vi "Write Shared Approved File Path.vi"(8 "error in":errorcluster, 10 "Shared Approved File Path":path, 11 "Namer With Shared Approved File in":refnum<class "Namer With Shared Approved File.lvclass">) -> (0 "error out":errorcluster, 3 "Namer With Shared Approved File out":refnum<class "Namer With Shared Approved File.lvclass">)   [LabVIEW 2020, in "Approval Tests.lvlib" / "Namer With Shared Approved File.lvclass"]
uses:
  Namer With Shared Approved File.lvclass
  Namer With Shared Approved File.lvclass/Namer With Shared Approved File.ctl
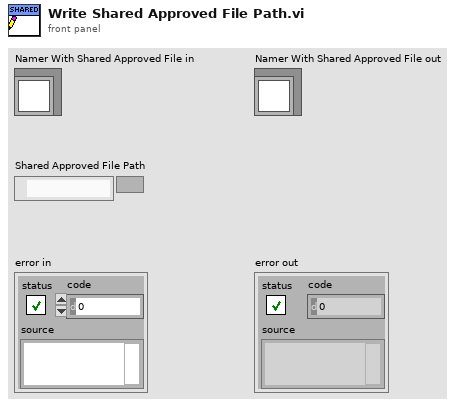
[diagram p1: front panel]
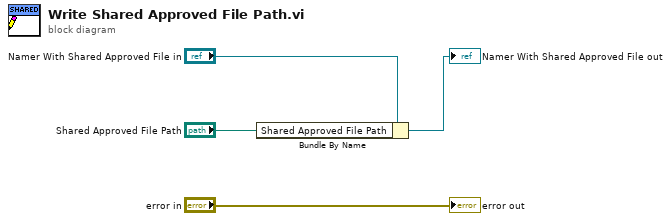
[diagram p0: block diagram]
diagram:
  n1 = Bundle By Name(cluster="Namer With Shared Approved File in", "Shared Approved File Path"="Shared Approved File Path") -> (→"Namer With Shared Approved File out":refnum<class "Namer With Shared Approved File.lvclass">)
  "error out" <- "error in"
